vi "Configure Output Range.vi"(7 "Range (0.0)":dbl format="%^.3e", 8 "error in (no error)":errorcluster {"code" format="%.0x"}, 9 "Range Type (1: Voltage)":i32(ring)=1 items=["Voltage"=1, "Current"=0], 10 "Channel Name (1)":string="1", 11 "VISA resource name":refnum<visa-resource-name>) -> (0 "error out":errorcluster {"code" format="%.0x"}, 3 "VISA resource name out":refnum<visa-resource-name>)   [LabVIEW 2018, in "Agilent N6700 Series.lvlib"]
doc: "Configures the power supply's output range on a channel. You specify whether you want to configure the voltage or current range, and the value to which to set the range.\n\n<b>Notes:</b>\n(1) Setting a voltage range can invalidate a previously configured current range.\n(2) Setting a current range can invalidate a previously configured voltage range."
uses:
  Agilent N6700 Series.lvlib
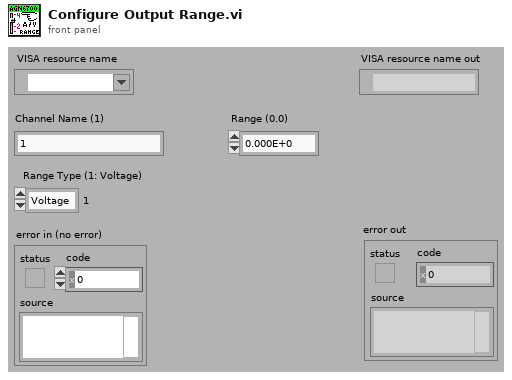
[diagram p1: front panel]
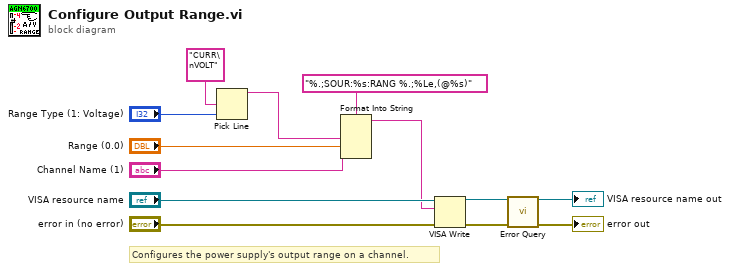
[diagram p0: block diagram]
diagram:
  # "Configures the power supply's output range on a channel."
  n1 = Pick Line(multi-line string="CURR\nVOLT", line index="Range Type (1: Voltage)") -> (output string=w8:string)  [unwired: 1 in]
  n2 = Format Into String(format string="%.;SOUR:%s:RANG %.;%Le,(@%s)", w8, "Range (0.0)", "Channel Name (1)") -> (resulting string=w5:string)  [unwired: 2 in, 1 out]
  n3 = VISA Write(VISA resource name="VISA resource name", write buffer=w5, error in (no error)="error in (no error)") -> (VISA resource name out=w2:refnum<visa-resource-name>, error out=w1:errorcluster)  [unwired: 1 out]
  n4 = call "Error Query.vi"("VISA resource name"=w2, "error in (no error)"=w1) -> ("VISA resource name out"=→"VISA resource name out":refnum<visa-resource-name>, "error out"=→"error out":errorcluster)  [unwired: 10 in, 2 out]
